vi "FPGA Debug (RT).vi"() -> ()   [LabVIEW 2013]
uses:
  <vilib>/FPGAPlugInAG/sbRIO-9626/niLvFpga_Open_sbRIO-9626.vi
  <vilib>/rvi/interface/common/niFpgaWaitOnOcc.vi
  <vilib>/Utility/error.llb/Error Cluster From Error Code.vi
  <vilib>/rvi/errors/niLvFpgaAdjustHostInterfaceError.vi
  <vilib>/rvi/interface/nirviOpenFPGA/nirviOpenFPGA.xnode
  FPGA Bitfiles/Gas Rack.lvbitx
  <vilib>/rvi/interface/nirviMethod/nirviMethod.xnode
  <vilib>/rvi/interface/nirviReadWriteControl/nirviReadWriteControl.xnode
  <vilib>/rvi/errors/niLvFpgaMergeErrorWithErrorCode.vi
  <vilib>/FPGAPlugInAG/sbRIO-9626/niLvFpga_ReadFifo_sbRIO-9626.vi
  <vilib>/ptbypt/NI_PtbyPt.lvlib
  NiFpgaLv.dll
panel:
  out "x-y":dbl
  in  "sample length":i32=5
  out "Speed 2":dbl
  out "Graph Percentile":sgl[][](graph)
  out "Graph Hold":sgl[][](graph)
  out "actual time":dbl
  in  "threshold level":fxp<+/-,24,7>
  in  "Hysteresis":fxp<+,10,6>
  out "DataCluster.Speed":dbl
  in  "BL Threshold":bool
  in  "PumpCt4rpm":bool
  out "Graph":sgl[][](graph)
  in  "CommSegs":i32
  in  "Update Graph":bool
  in  "PresCtrl":fxp<+/-,20,5>
  in  "VoltCtrl":fxp<+/-,20,5>
  in  "PSenable":bool
  in  "Graph Refresh (s)":dbl
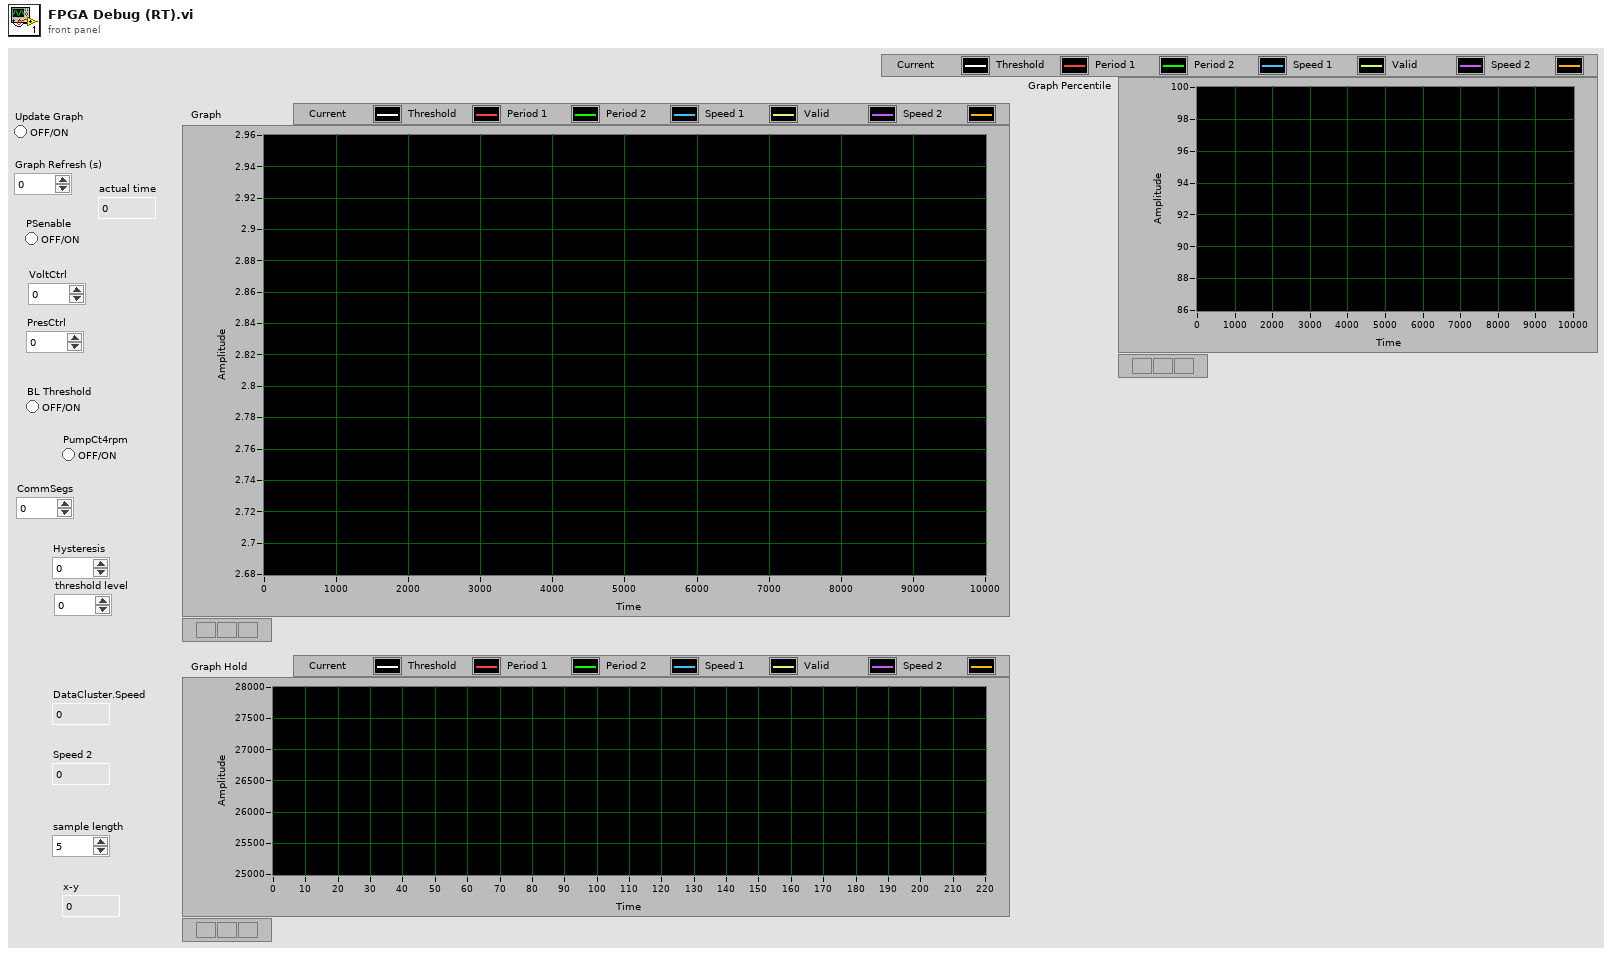
[diagram p1: front panel]
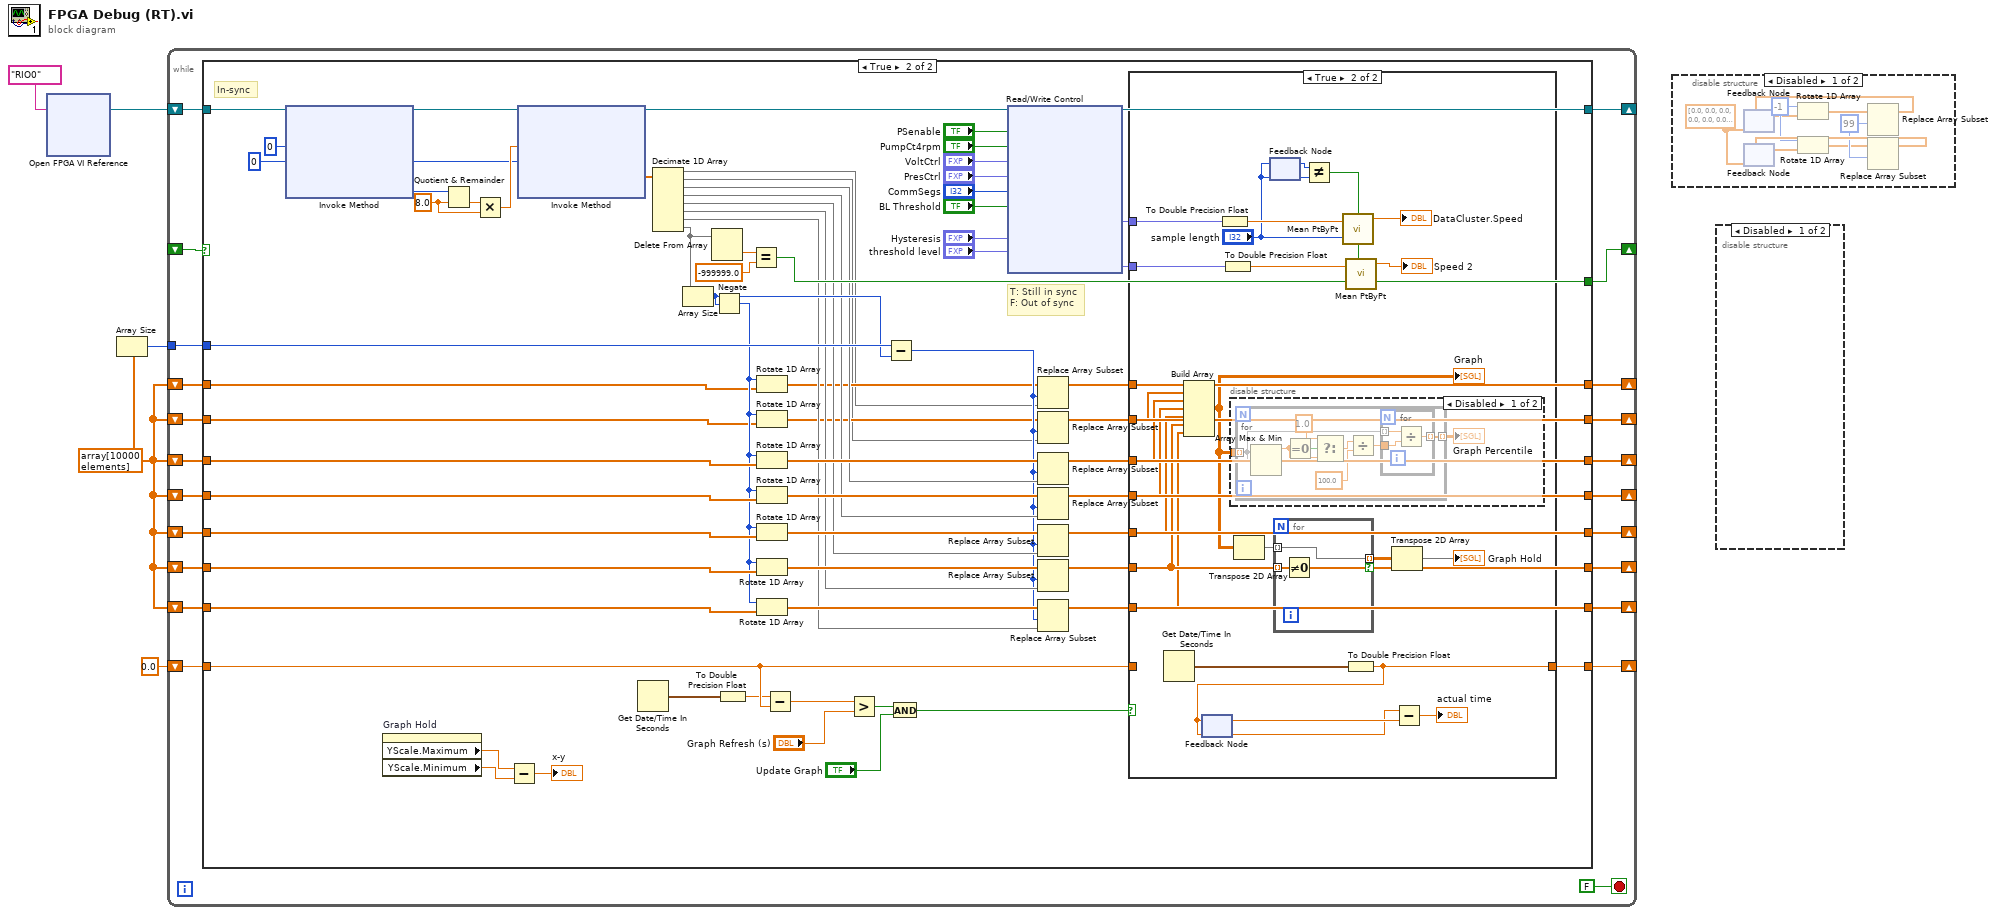
[diagram p0: block diagram]
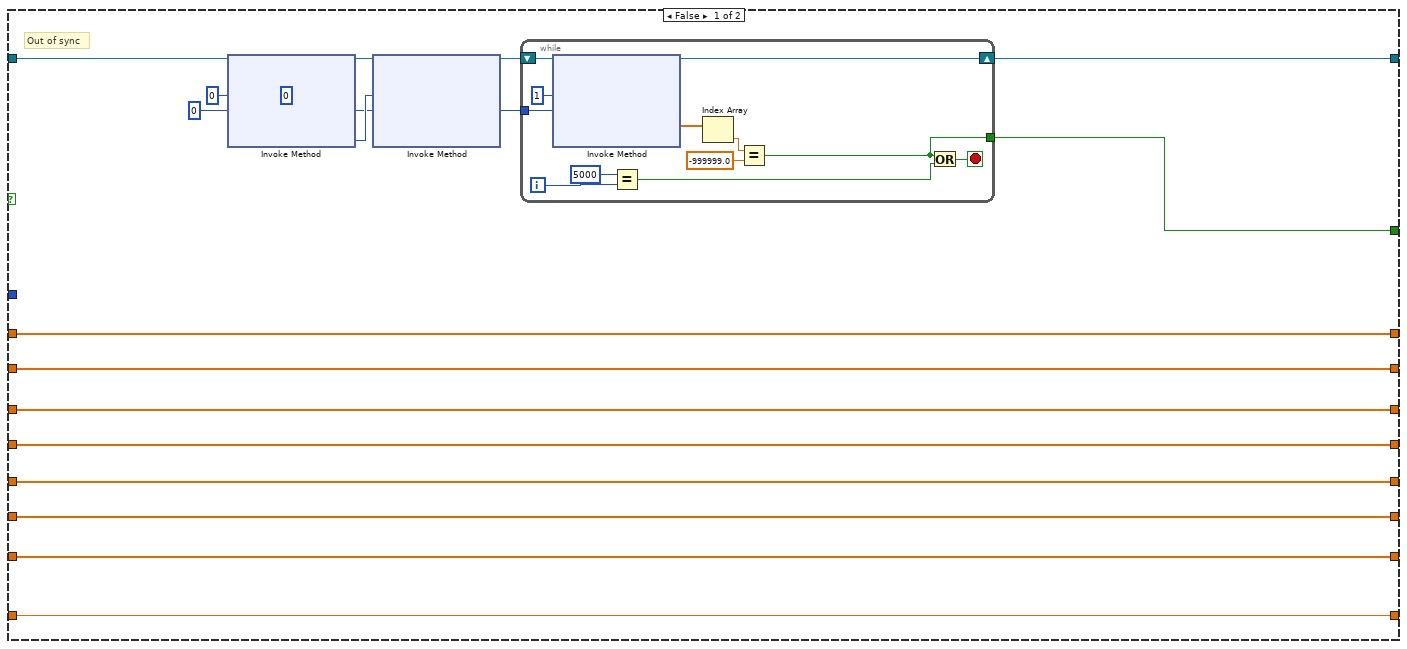
[diagram p4: hidden frame]
diagram:
  w1 = sgl[] array[10000 elements]
  n1 = xnode "Open FPGA VI Reference"("resource name"=tag "RIO0") -> ("FPGA VI Reference Out"=w5:refnum<k20>)  [unwired: 1 in, 1 out]
  n2 = Array Size(array=w1) -> (size(s)=w2:i32)
  n3 = while {
    shift-right: [w19] -> _
    shift-left: w5 -> [w26]
    shift-right: [w24] -> _
    shift-left: _ -> [w27]
    shift-right: [w22] -> _
    shift-left: w1 -> [w23]
    shift-right: [w21] -> _
    shift-left: 0.0 -> [w20]
    shift-right: [w18] -> _
    shift-left: w1 -> [w14]
    shift-right: [w17] -> _
    shift-left: w1 -> [w13]
    shift-right: [w16] -> _
    shift-left: w1 -> [w12]
    shift-right: [w15] -> _
    shift-left: w1 -> [w11]
    tunnel: w2 -> [w10]
    shift-right: [w9] -> _
    shift-left: w1 -> [w6]
    shift-right: [w8] -> _
    shift-left: w1 -> [w7]
    stop <- FALSE stop-if-true
    n4 = case shown="True" w27 {
      tunnel: w26 -> [w42 w117]
      tunnel: [w38 w120] -> w24
      tunnel: w23 -> [w37 w119]
      tunnel: [w37 w93] -> w22
      tunnel: [w36 w112] -> w21
      tunnel: w20 -> [w36 w110]
      tunnel: [w34 w70] -> w19
      tunnel: [w33 w92] -> w18
      tunnel: [w32 w91] -> w17
      tunnel: [w31 w90] -> w16
      tunnel: [w30 w89] -> w15
      tunnel: w14 -> [w33 w97]
      tunnel: w13 -> [w32 w96]
      tunnel: w12 -> [w31 w95]
      tunnel: w11 -> [w30 w94]
      tunnel: w10 -> [_ w80]
      tunnel: [w28 w59] -> w9
      tunnel: [w29 w60] -> w8
      tunnel: w7 -> [w29 w62]
      tunnel: w6 -> [w28 w61]
      frame False {
        w35 = 0 ("Timeout (ms)")
        (unwired) u32 0 ("Number of Elements")
        # "Out of sync"
        n5 = xnode "Invoke Method"("FPGA VI Reference In"=w42, "Number of Elements"=u32 0, "Timeout (ms)"=w35) -> ("FPGA VI Reference Out"=w41:refnum<k20>, "Elements Remaining"=w40:u32)  [unwired: 1 in, 2 out]
        n6 = xnode "Invoke Method"("FPGA VI Reference In"=w41, "Number of Elements"=w40, "Timeout (ms)"=w35) -> ("FPGA VI Reference Out"=w39:refnum<k20>)  [unwired: 1 in, 3 out]
        n7 = while {
          shift-right: [w46] -> w34
          shift-left: w39 -> [w55]
          tunnel: [w45] -> w38
          tunnel: w35 -> [w44]
          i -> [w50]
          stop <- w47 stop-if-true
          n8 = xnode "Invoke Method"("FPGA VI Reference In"=w55, "Number of Elements"=u32 1, "Timeout (ms)"=w44) -> ("FPGA VI Reference Out"=w46:refnum<k20>, "Data"=w53:sgl[])  [unwired: 1 in, 2 out]
          n9 = Equal?(x=5000, y=w50) -> (x = y?=w48:bool)
          n10 = Index Array(array=w53) -> (element=w52:sgl)  [unwired: 1 in]
          n11 = Equal?(x=w52, y=sgl -999999.0) -> (x = y?=w45:bool)
          n12 = Or(x=w45, y=w48) -> (x .or. y?=w47:bool)
        }
      }
      frame True {
        w107 = 0 ("Timeout (ms)")
        w123 = 8.0 ("y")
        # "T: Still in sync\nF: Out of sync"
        # "In-sync"
        n13 = xnode "Invoke Method"("FPGA VI Reference In"=w117, "Number of Elements"=u32 0, "Timeout (ms)"=w107) -> ("FPGA VI Reference Out"=w114:refnum<k20>, "Elements Remaining"=w116:u32)  [unwired: 1 in, 2 out]
        n14 = property on="Graph Hold" class="WFGraph (strict)"() -> ("YScale.Maximum"=w58:dbl, "YScale.Minimum"=w57:dbl)  [unwired: 2 in, 2 out]
        n15 = Quotient & Remainder(x=w116, y=w123) -> (floor(x/y)=w124:dbl)  [unwired: 1 out]
        n16 = Multiply(x=w124, y=w123) -> (x*y=w115:dbl)
        n17 = Subtract(x=w58, y=w57) -> (x-y=→"x-y":dbl)
        n18 = xnode "Invoke Method"("FPGA VI Reference In"=w114, "Number of Elements"=w115, "Timeout (ms)"=w107) -> ("FPGA VI Reference Out"=w82:refnum<k20>, "Data"=w113:sgl[])  [unwired: 1 in, 2 out]
        n19 = Get Date/Time In Seconds() -> (seconds since 1Jan1904=w111:timestamp)
        n20 = Decimate 1D Array(w113) -> (w63:sgl[], w64:sgl[], w74:sgl[], w75:sgl[], w76:sgl[], w77:sgl[], w78:sgl[], w102:sgl[])
        n21 = Array Size(array=w102) -> (size(s)=w79:i32)
        n22 = Delete From Array(array=w102) -> (deleted portion=w121:sgl)  [unwired: 2 in, 1 out]
        n23 = Negate(x=w79) -> (-x=w68:i32)
        n24 = To Double Precision Float(number=w111) -> (double precision float=w71:dbl)
        n25 = Equal?(x=w121, y=sgl -999999.0) -> (x = y?=w120:bool)
        n26 = Rotate 1D Array(1:w61, 2:w68) -> (0:w66:sgl[])
        n27 = Rotate 1D Array(1:w62, 2:w68) -> (0:w65:sgl[])
        n28 = Rotate 1D Array(1:w119, 2:w68) -> (0:w118:sgl[])
        n29 = Rotate 1D Array(1:w97, 2:w68) -> (0:w101:sgl[])
        n30 = Rotate 1D Array(1:w96, 2:w68) -> (0:w100:sgl[])
        n31 = Rotate 1D Array(1:w95, 2:w68) -> (0:w99:sgl[])
        n32 = Rotate 1D Array(1:w94, 2:w68) -> (0:w98:sgl[])
        n33 = Subtract(x=w71, y=w110) -> (x-y=w109:dbl)
        n34 = Greater?(x=w109, y="Graph Refresh (s)") -> (0:w105:bool)
        n35 = Subtract(x=w80, y=w79) -> (x-y=w67:i32)
        n36 = And(x=w105, y="Update Graph") -> (x .and. y?=w103:bool)
        n37 = xnode "Read/Write Control"("FPGA VI Reference In"=w82, "PSenable"="PSenable", "PumpCt4rpm"="PumpCt4rpm", "VoltCtrl"="VoltCtrl", "PresCtrl"="PresCtrl", "CommSegs"="CommSegs", "BL Threshold"="BL Threshold", "Hysteresis"="Hysteresis", "threshold level"="threshold level") -> ("FPGA VI Reference Out"=w70:refnum<k20>, "DataCluster.Speed"=w81:fxp<+/-,25,15>, "Speed 2"=w69:fxp<+/-,38,38>)  [unwired: 1 in, 1 out]
        n38 = Replace Array Subset(array=w66, new element=w63, index=w67) -> (w59:sgl[])
        n39 = Replace Array Subset(array=w65, new element=w64, index=w67) -> (w60:sgl[])
        n40 = Replace Array Subset(array=w118, new element=w74, index=w67) -> (w93:sgl[])
        n41 = Replace Array Subset(array=w101, new element=w75, index=w67) -> (w92:sgl[])
        n42 = Replace Array Subset(array=w100, new element=w76, index=w67) -> (w91:sgl[])
        n43 = Replace Array Subset(array=w99, new element=w77, index=w67) -> (w90:sgl[])
        n44 = Replace Array Subset(array=w98, new element=w78, index=w67) -> (w89:sgl[])
        n45 = case shown="True" w103 {
          tunnel: [w125 w142] -> w112
          tunnel: w110 -> [w125 _]
          tunnel: w93 -> [_ w148]
          tunnel: w92 -> [_ w145]
          tunnel: w91 -> [_ w147]
          tunnel: w90 -> [_ w138]
          tunnel: w89 -> [_ w146]
          tunnel: w81 -> [_ w133]
          tunnel: w69 -> [_ w130]
          tunnel: w60 -> [_ w140]
          tunnel: w59 -> [_ w141]
          frame False {
          }
          frame True {
            n46 = Get Date/Time In Seconds() -> (seconds since 1Jan1904=w149:timestamp)
            n47 = Build Array(w141, w140, w148, w145, w147, w138, w146) -> (w139:sgl[][])
            "Graph" <- w139
            n48 = To Double Precision Float(number=w133) -> (double precision float=w134:dbl)
            n49 = To Double Precision Float(number=w130) -> (double precision float=w131:dbl)
            n50 = disable-structure shown="Disabled" {
              disable-tunnel: w139 -> [w153 _]
              frame Disabled {
                n51 = for {
                  tunnel: w153 -> [w162] mode=indexing
                  tunnel: [w159] -> w154 mode=indexing
                  n52 = Array Max & Min(array=w162) -> (max value=w157:sgl)  [unwired: 3 out]
                  n53 = Equal To 0?(x=w157) -> (x = 0?=w158:bool)
                  n54 = Select(t=sgl 1.0, s=w158, f=w157) -> (s? t:f=w156:sgl)
                  n55 = Divide(x=w156, y=sgl 100.0) -> (x/y=w160:sgl)
                  n56 = for {
                    tunnel: w162 -> [w165] mode=indexing
                    tunnel: w160 -> [w164]
                    tunnel: [w163] -> w159 mode=indexing
                    n57 = Divide(x=w165, y=w164) -> (x/y=w163:sgl)
                  }
                }
                "Graph Percentile" <- w154
              }
              frame Enabled {
              }
            }
            n58 = Transpose 2D Array(2D array=w139) -> (transposed array=w135:sgl[][])
            n59 = feedback-in #1("sample length") -> ()
            n60 = feedback #1("sample length") -> (w128:i32)
            n61 = for {
              tunnel: w135 -> [w151] mode=indexing
              tunnel: [w151] -> w137 mode=indexing if=w150
              tunnel: w138 -> [w152] mode=indexing
              n62 = Not Equal To 0?(x=w152) -> (x != 0?=w150:bool)
            }
            n63 = Not Equal?(x=w128, y="sample length") -> (x != y?=w126:bool)
            n64 = call <vilib>:"Mean PtByPt.vi"("x"=w134, "sample length"="sample length", "initialize"=w126) -> ("mean"=→"DataCluster.Speed":dbl)  [unwired: 1 in, 1 out]
            n65 = call <vilib>:"Mean PtByPt.vi"("x"=w131, "initialize"=w126) -> ("mean"=→"Speed 2":dbl)  [unwired: 2 in, 1 out]
            n66 = To Double Precision Float(number=w149) -> (double precision float=w142:dbl)
            n67 = feedback #2(w142) -> (w143:dbl)
            n68 = feedback-in #2(w142) -> ()
            n69 = Transpose 2D Array(2D array=w137) -> (transposed array=→"Graph Hold":sgl[][])
            n70 = Subtract(x=w142, y=w143) -> (x-y=→"actual time":dbl)
          }
        }
      }
    }
  }
  n71 = disable-structure shown="Disabled" {
    frame Disabled {
      w172 = 99 ("index")
      w169 = -1 ("n")
      w166 = dbl[] [0.0, 0.0, 0.0, 0.0, 0.0, 0.0, 0.0, 0.0, 0.0, 0.0, 0.0, 0.0, 0.0, 0.0, 0.0, 0.0, 0.0, 0.0, 0.0, 0.0, 0.0, 0.0, 0.0, 0.0, 0.0, 0.0, 0.0, 0.0, 0.0, 0.0, 0.0, 0.0, 0.0, 0.0, 0.0, 0.0, 0.0, 0.0, 0.0, 0.0, 0.0, 0.0, 0.0, 0.0, 0.0, 0.0, 0.0, 0.0, 0.0, 0.0, 0.0, 0.0, 0.0, 0.0, 0.0, 0.0, 0.0, 0.0, 0.0, 0.0, 0.0, 0.0, 0.0, 0.0, 0.0, 0.0, 0.0, 0.0, 0.0, 0.0, 0.0, 0.0, 0.0, 0.0, 0.0, 0.0, 0.0, 0.0, 0.0, 0.0, 0.0, 0.0, 0.0, 0.0, 0.0, 0.0, 0.0, 0.0, 0.0, 0.0, 0.0, 0.0, 0.0, 0.0, 0.0, 0.0, 0.0, 0.0, 0.0, 0.0]
      n72 = feedback #3(w166) -> (w167:dbl[])
      n73 = feedback #4(w166) -> (w168:dbl[])
      n74 = Rotate 1D Array(1:w167, 2:w169) -> (0:w171:dbl[])
      n75 = Rotate 1D Array(1:w168, 2:w169) -> (0:w170:dbl[])
      n76 = Replace Array Subset(array=w171, index=w172) -> (w173:dbl[])  [unwired: 1 in]
      n77 = feedback-in #3(w173) -> ()
      n78 = Replace Array Subset(array=w170, index=w172) -> (w174:dbl[])  [unwired: 1 in]
      n79 = feedback-in #4(w174) -> ()
    }
    frame Enabled {
    }
  }
  n80 = disable-structure shown="Disabled" {
    frame Disabled {
    }
    frame Enabled {
    }
  }
